vi "Initialize Devices.vi"(8 "error in (no error)":errorcluster, 11 "Starter Kit host FPGA 1.0 in":refnum<class "NI_Robotics_Starter Kit Host_FPGA_1.0.lvclass">) -> (0 "error out":errorcluster, 3 "Starter Kit host FPGA 1.0 out":refnum<class "NI_Robotics_Starter Kit Host_FPGA_1.0.lvclass">)   [LabVIEW 2017, in "NI_Robotics_Starter Kit Host_FPGA_1.0.lvclass"]
uses:
  <vilib>/robotics/Starter Kit/1.0/FPGA Host Interface/NI_Robotics_Starter Kit Host_FPGA_1.0.lvclass
  c:/Program Files (x86)/National Instruments/LabVIEW 2017/vi.lib/robotics/Starter Kit/Host Interface/NI_Robotics_Starter Kit Host.lvclass
  <vilib>/robotics/Starter Kit/1.0/FPGA Host Interface/NI_Robotics_Starter Kit Host_FPGA_1.0.lvclass/NI_Robotics_Starter Kit Host_FPGA_1.0.ctl
  <vilib>/robotics/Starter Kit/Host Interface/NI_Robotics_Starter Kit Host.lvclass/NI_Robotics_Starter Kit Host.ctl
  <vilib>/robotics/Starter Kit/FPGA Direct IO/NI_Robotics_Starter Kit Direct IO_FPGA.lvclass/NI_Robotics_Starter Kit Direct IO_FPGA.ctl
  <vilib>/robotics/Starter Kit/Base Device/NI_Robotics_Starter Kit Base Device.lvclass/NI_Robotics_Starter Kit Base Device.ctl
  <vilib>/robotics/Starter Kit/Servo Motor 1.0/NI_Robotics_Starter Kit Servo Motor_1.0.lvclass
  c:/Program Files (x86)/National Instruments/LabVIEW 2017/vi.lib/robotics/Starter Kit/Servo Motor/NI_Robotics_Starter Kit Servo Motor.lvclass
  <vilib>/robotics/Starter Kit/FPGA Direct IO/NI_Robotics_Starter Kit Direct IO_FPGA.lvclass
  c:/Program Files (x86)/National Instruments/LabVIEW 2017/vi.lib/robotics/Starter Kit/Base Device/NI_Robotics_Starter Kit Base Device.lvclass
  c:/Program Files (x86)/National Instruments/LabVIEW 2017/vi.lib/robotics/Starter Kit/Direct IO/NI_Robotics_Starter Kit Direct IO.lvclass
  <vilib>/robotics/Starter Kit/Host Interface/NI_Robotics_Starter Kit Host.lvclass
  <instrlib>/DC Motor Controller/HAIOL/FPGA/DC Motor Controller FPGA.lvclass
  <instrlib>/Parallax PING)))/HAIOL/FPGA/Parallax PING))) FPGA.lvclass
  <instrlib>/Parallax Standard Servo/HAIOL/FPGA/Parallax Standard Servo FPGA.lvclass
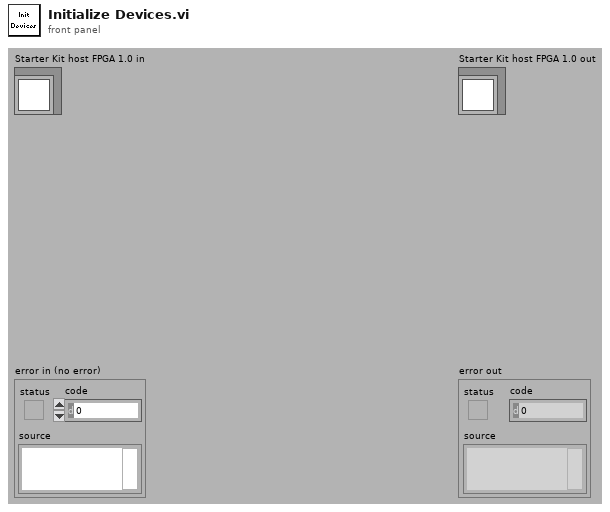
[diagram p1: front panel]
types:
  T1 = typedef "NI_Robotics_Starter Kit Host_FPGA_1.0.lvclass/FPGA Refnum.ctl" = refnum<k20>
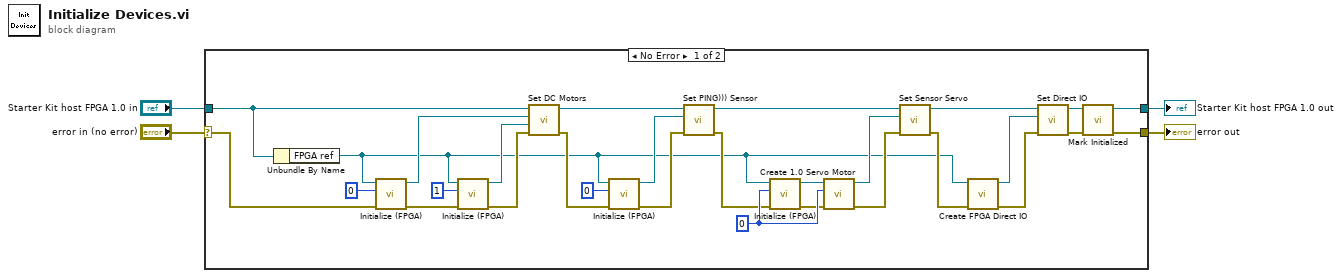
[diagram p0: block diagram]
diagram:
  n1 = case shown="No Error" "error in (no error)" {
    selector: "error in (no error)" -> [w5 w35]
    tunnel: [w6 w35] -> w3
    tunnel: [w7 w34] -> w1
    tunnel: "Starter Kit host FPGA 1.0 in" -> [w8 w34]
    frame No Error {
      w32 = 0 ("servo ID")
      n2 = Unbundle By Name(w8) -> ("FPGA ref"=w9:T1)
      n3 = call <instrlib>:"Initialize (FPGA).vi"("error in (no error)"=w5, "Actuator ID (0)"=u16 0 ("motor ID"), "FPGA VI Reference"=w9) -> ("error out"=w25:errorcluster, "DC Motor Controller out"=w22:refnum<class "DC Motor Controller.lvclass">)  [unwired: 7 in]
      n4 = call <instrlib>:"Initialize (FPGA).vi"("error in (no error)"=w25, "Actuator ID (0)"=u16 1 ("motor ID"), "FPGA VI Reference"=w9) -> ("error out"=w20:errorcluster, "DC Motor Controller out"=w21:refnum<class "DC Motor Controller.lvclass">)  [unwired: 7 in]
      n5 = call <vilib>:"Set DC Motors.vi"("error in (no error)"=w20, "DC motor 1 (right)"=w21, "DC motor 0 (left)"=w22, "NI_Robotics_Starter Kit Host in"=w8) -> ("error out"=w18:errorcluster, "NI_Robotics_Starter Kit Host out"=w17:refnum<class "NI_Robotics_Starter Kit Host_FPGA_1.0.lvclass">)  [unwired: 6 in]
      n6 = call <instrlib>:"Initialize (FPGA).vi"("error in (no error)"=w18, "Sensor ID (0)"=0 ("PING))) ID"), "FPGA VI Reference"=w9) -> ("error out"=w15:errorcluster, "Parallax PING))) out"=w16:refnum<class "Parallax PING))).lvclass">)  [unwired: 7 in]
      n7 = call <vilib>:"Set PING))) Sensor.vi"("error in (no error)"=w15, "PING)))"=w16, "NI_Robotics_Starter Kit Host in"=w17) -> ("error out"=w28:errorcluster, "NI_Robotics_Starter Kit Host out"=w14:refnum<class "NI_Robotics_Starter Kit Host_FPGA_1.0.lvclass">)  [unwired: 7 in]
      n8 = call <instrlib>:"Initialize (FPGA).vi"("error in (no error)"=w28, "Actuator ID (0)"=w32, "FPGA VI Reference"=w9) -> ("error out"=w31:errorcluster, "Parallax Standard Servo out"=w29:refnum<class "Parallax Standard Servo.lvclass">)  [unwired: 7 in]
      n9 = call <vilib>:"Create 1.0 Servo Motor.vi"("error in (no error)"=w31, "servo ID"=w32, "Parallax standard servo"=w29) -> ("error out"=w33:errorcluster, "Starter Kit Servo Motor_1.0 out"=w30:refnum<class "NI_Robotics_Starter Kit Servo Motor_1.0.lvclass">)  [unwired: 7 in]
      n10 = call <vilib>:"Set Sensor Servo.vi"("error in (no error)"=w33, "sensor servo"=w30, "NI_Robotics_Starter Kit Host in"=w14) -> ("error out"=w13:errorcluster, "NI_Robotics_Starter Kit Host out"=w12:refnum<class "NI_Robotics_Starter Kit Host_FPGA_1.0.lvclass">)  [unwired: 7 in]
      n11 = call <vilib>:"Create FPGA Direct IO.vi"("error in (no error)"=w13, "FPGA Interface"=w9) -> ("error out"=w10:errorcluster, "FPGA direct IO out"=w11:refnum<class "NI_Robotics_Starter Kit Direct IO_FPGA.lvclass">)  [unwired: 8 in]
      n12 = call <vilib>:"Set Direct IO.vi"("error in (no error)"=w10, "direct IO"=w11, "NI_Robotics_Starter Kit Host in"=w12) -> ("error out"=w27:errorcluster, "NI_Robotics_Starter Kit Host out"=w26:refnum<class "NI_Robotics_Starter Kit Host_FPGA_1.0.lvclass">)  [unwired: 7 in]
      n13 = call <vilib>:"Mark Initialized.vi"("error in (no error)"=w27, "starter kit host in"=w26) -> ("error out"=w6:errorcluster, "starter kit host out"=w7:refnum<class "NI_Robotics_Starter Kit Host_FPGA_1.0.lvclass">)  [unwired: 8 in]
    }
    frame Error {
    }
  }
  "error out" <- w3
  "Starter Kit host FPGA 1.0 out" <- w1
